vi "Report1.vi"(6 "文件重命名":bool, 7 "文件名称":string, 8 "错误输入（无错误）":errorcluster, 11 "检测结果":bool[][](array[boolean])=[[TRUE]]) -> (0 "error out":errorcluster caption="错误输出", 3 "PRODUCT_VAULE":string)   [LabVIEW 2020]
uses:
  Global_Variable/Global.vi
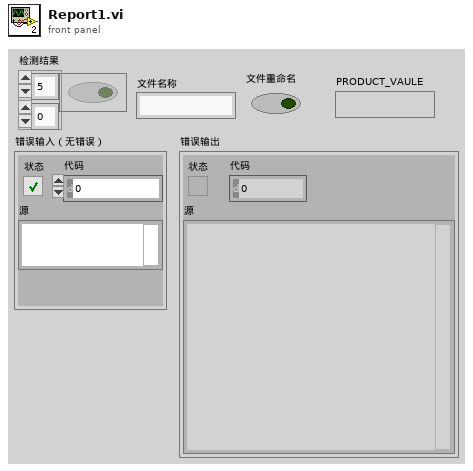
[diagram p1: front panel]
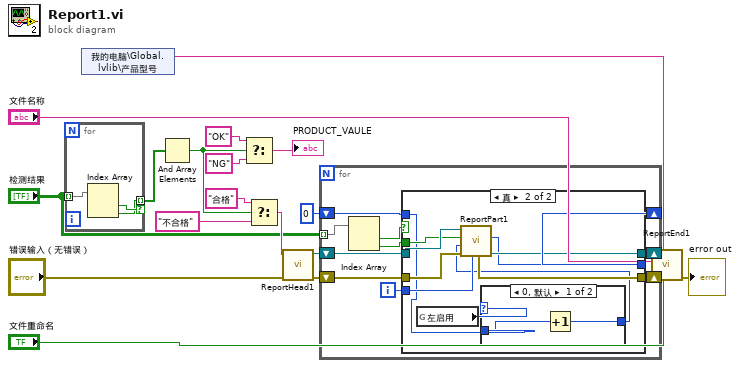
[diagram p0: block diagram]
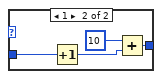
[diagram p3: hidden frame]
diagram:
  n1 = for {
    tunnel: [w20] -> w4 mode=indexing if=w21
    tunnel: "检测结果" -> [w22] mode=indexing
    n2 = Index Array(array=w22) -> (element #1=w21:bool, element #2=w20:bool)  [unwired: 2 in]
  }
  n3 = shared-variable "我的电脑\\Global.lvlib\\产品型号"() -> (w1:string)  [unwired: 1 in, 1 out]
  n4 = And Array Elements(Boolean array=w4) -> (logical AND=w5:bool)
  n5 = Select(t="OK", s=w5, f="NG") -> (s? t:f=→"PRODUCT_VAULE":string)
  n6 = Select(t="合格", s=w5, f="不合格") -> (s? t:f=w10:string)
  n7 = call "ReportHead1.vi"("error in (no error)"="错误输入（无错误）", "产品状态"=w10) -> ("error out"=w18:errorcluster, "report out"=w19:refnum<class "NI_report.lvclass">)  [unwired: 8 in]
  n8 = for {
    shift-right: [w30] -> w17
    shift-left: w19 -> [w32]
    shift-right: [w29] -> w16
    shift-left: w18 -> [w31]
    tunnel: "检测结果" -> [w25] mode=indexing
    shift-right: [w26] -> _
    shift-left: 0 ("索引OUT") -> [w27]
    i -> [w28]
    n9 = Index Array(array=w25) -> (element #1=w24:bool, element #2=w23:bool)  [unwired: 2 in]
    n10 = case shown="真" w24 {
      tunnel: w32 -> [w34 w43]
      tunnel: w31 -> [w35 w44]
      tunnel: [w34 w42] -> w30
      tunnel: [w35 w40] -> w29
      tunnel: w28 -> [_ w45]
      tunnel: w23 -> [_ w39]
      tunnel: w27 -> [w33 w37]
      tunnel: [w33 w41] -> w26
      frame False {
      }
      frame True {
        n11 = global read "Global.vi" "左启用"() -> (w38:i16)
        n12 = case shown="0, 默认" w38 {
          tunnel: w37 -> [w47 w51]
          tunnel: [w46 w50] -> w36
          frame 0, Default {
            n13 = Increment(x=w47) -> (x+1=w46:i32)
          }
          frame 1 {
            n14 = Increment(x=w51) -> (x+1=w49:i32)
            n15 = Add(x=10, y=w49) -> (x+y=w50:i32)
          }
        }
        n16 = call "ReportPart1.vi"("试验项目"=w45, "error in"=w44, "索引IN"=w36, "合格"=w39, "report in"=w43) -> ("error out 2"=w40:errorcluster, "索引OUT"=w41:i32, "report out"=w42:refnum<class "NI_report.lvclass">)  [unwired: 4 in]
      }
    }
  }
  n17 = call "ReportEnd1.vi"("文件重命名"="文件重命名", "产品型号"=w1, "error in (no error)"=w16, "文件名称"="文件名称", "report in"=w17) -> ("error out"=→"error out":errorcluster)  [unwired: 6 in]
